vi "AB_Engine_RESTful_Verify_Configuration.vi"(6 "destinations":refnum<class "AB_Destination.lvclass">[](array[class]), 7 "path":path, 8 "error in (no error)":errorcluster, 10 "flat file layout":bool, 11 "sourceItems":refnum<class "AB_Source.lvclass">[](array[class])) -> (0 "error out":errorcluster, 1 "viConfigs":T1[](array[typedef]), 4 "relative VI paths":path[](array[path]))   [LabVIEW 2020]
uses:
  <vilib>/AppBuilder/AB_Classes/Source/AB_Source.lvclass
  <vilib>/AppBuilder/AB_Classes/Source/RESTfulVI/Configure_RESTfulVI/AB_RESTful_Configuration.ctl
  <vilib>/AppBuilder/AB_Classes/Source/RESTfulVI/Configure_RESTfulVI/AB_RESTful_VIType.ctl
  <vilib>/AppBuilder/AB_Classes/Source/RESTfulVI/Configure_RESTfulVI/AB_RESTful_OutputType.ctl
  <vilib>/AppBuilder/AB_Classes/Source/RESTfulVI/Configure_RESTfulVI/AB_RESTful_OutputFormat.ctl
  <vilib>/AppBuilder/AB_Classes/Destination/AB_Destination.lvclass
  <vilib>/AppBuilder/AB_Classes/Source/RESTfulVI/AB_Source_RESTfulVI.lvclass
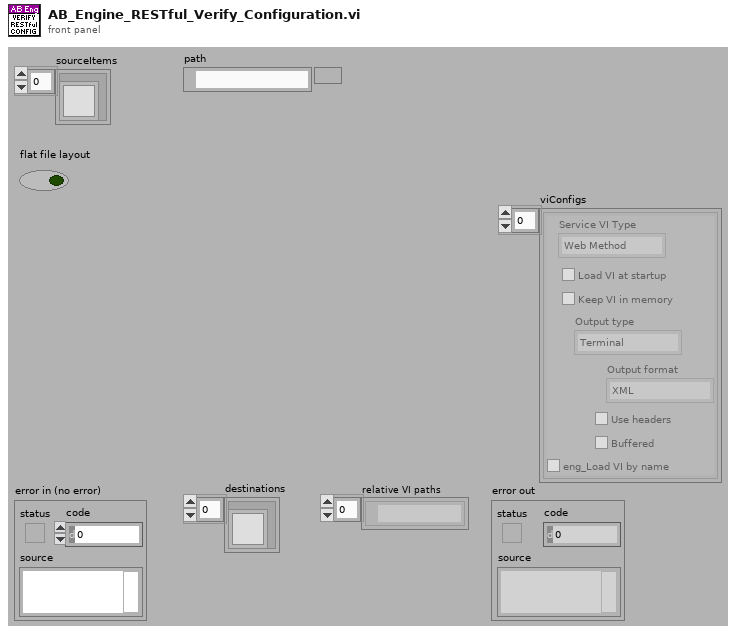
[diagram p1: front panel]
types:
  T1 = typedef "AB_RESTful_Configuration.ctl" = cluster{"Service VI Type":T2, "Load VI at statup":bool, "Keep VI in memory":bool, "Output type":T3, "Output format":T4, "Use headers":bool, "Buffered":bool, "eng_Load VI by name":bool}
  T2 = typedef "AB_RESTful_VIType.ctl" = enum32{"Web Method", "Auxiliary", "eng_Internal", "eng_Content"}
  T3 = typedef "AB_RESTful_OutputType.ctl" = enum32{"Terminal", "Stream"}
  T4 = typedef "AB_RESTful_OutputFormat.ctl" = enum32{"XML", "Text", "HTML", "JSON"}
  T5 = typedef "AB_Source.ctl" = cluster{"path":path, "itemID":string, "parentIndex":i32, "sourceInclusion":T6, "destinationIndex":i32, "properties":T7[], "newName":string, "lvfile":bool, "valid":bool, "eng_inBuild":bool, "eng_isNonVILink":bool, "Amalgamation":bool, "Amalgamation Piece":bool, "eng_delimitedName":string, "preventRename":bool}
  T6 = typedef "AB_Source_Inclusion.ctl" = enum16{"IncludeIfReferenced", "Include", "Exclude", "TopLevel"}
  T7 = typedef "AB_Source_Properties.ctl" = cluster{"sourcePropertyType":T8, "value":variant}
  T8 = typedef "AB_Source_Property_Type.ctl" = enum16{"Remove block diagram", "Remove front panel", "Password", "Window has title bar", "Show menu bar", "Show vertical scroll bar", "Show horizontal scroll bar", "Show toolbar", "Show Abort button", "Show fp when called", "Window behavior", "Allow user to close window", "Window run-time position", "Run when opened", "Allow debugging", "Auto error handling", "Generate guard code", "Use stack variables", "Expression folding", "Integer only", "Inline subVI"}
  T9 = typedef "AB_Destination.ctl" = cluster{"destName":string, "path":path, "libraryName":string, "preserveHierarchy":bool, "eng_inBuild":bool, "eng_libraryReference":refnum<vi>, "eng_restictAddToNewLibrary":bool}
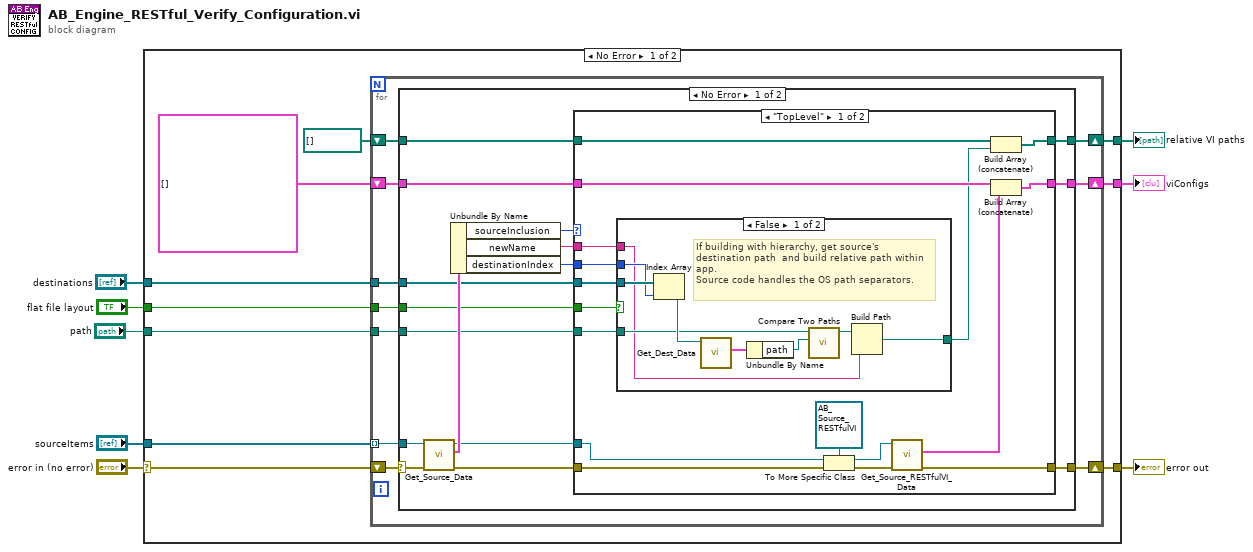
[diagram p0: block diagram]
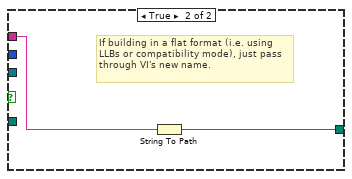
[diagram p2: hidden frame]
diagram:
  n1 = case shown="No Error" "error in (no error)" {
    selector: "error in (no error)" -> [w17 w79]
    tunnel: [w16 w79] -> w7
    tunnel: "sourceItems" -> [w18 _]
    tunnel: [w14 _] -> w5
    tunnel: "flat file layout" -> [w13 _]
    tunnel: "destinations" -> [w12 _]
    tunnel: "path" -> [w11 _]
    tunnel: [w9 _] -> w1
    frame No Error {
      n2 = for {
        tunnel: w18 -> [w28] mode=indexing
        shift-right: [w27] -> w16
        shift-left: w17 -> [w26]
        shift-right: [w25] -> w14
        shift-left: T1[] [] -> [w24]
        tunnel: w13 -> [w23]
        tunnel: w12 -> [w22]
        tunnel: w11 -> [w21]
        shift-right: [w20] -> w9
        shift-left: path[] [] -> [w19]
        n3 = case shown="No Error" w26 {
          selector: w26 -> [w37 w78]
          tunnel: w28 -> [w40 _]
          tunnel: [w38 w78] -> w27
          tunnel: [w36 w77] -> w25
          tunnel: w24 -> [w35 w77]
          tunnel: w23 -> [w34 _]
          tunnel: w22 -> [w32 _]
          tunnel: w21 -> [w31 _]
          tunnel: [w30 w76] -> w20
          tunnel: w19 -> [w29 w76]
          frame No Error {
            n4 = call <vilib>:"Get_Source_Data.vi"("error in (no error)"=w37, "Class in"=w40) -> ("error out"=w39:errorcluster, "data"=w44:T5, "Class out"=w41:refnum<class "AB_Source.lvclass">)  [unwired: 7 out]
            n5 = Unbundle By Name(w44) -> ("sourceInclusion"=w43:T6, "newName"=w42:string, "destinationIndex"=w33:i32)
            n6 = case shown="\"TopLevel\"" w43 {
              tunnel: w42 -> [w48 _]
              tunnel: w41 -> [w60 _]
              tunnel: w39 -> [w57 w75]
              tunnel: [w56 w75] -> w38
              tunnel: [w59 w74] -> w36
              tunnel: w35 -> [w58 w74]
              tunnel: w34 -> [w53 _]
              tunnel: w33 -> [w54 _]
              tunnel: w32 -> [w52 _]
              tunnel: w31 -> [w51 _]
              tunnel: [w46 w73] -> w30
              tunnel: w29 -> [w45 w73]
              frame "TopLevel" {
                n7 = case shown="False" w53 {
                  tunnel: w48 -> [w63 w72]
                  tunnel: [w62 w71] -> w47
                  tunnel: w52 -> [w70 _]
                  tunnel: w51 -> [w66 _]
                  tunnel: w54 -> [w69 _]
                  frame False {
                    # "If building with hierarchy, get source's destination path  and build relative path within app. \nSource code handles the OS path separators."
                    n8 = Index Array(array=w70, index=w69) -> (element=w68:refnum<class "AB_Destination.lvclass">)
                    n9 = call <vilib>:"Get_Dest_Data.vi"("Class in"=w68) -> ("destName"=w67:T9)  [unwired: 1 in, 9 out]
                    n10 = Unbundle By Name(w67) -> ("path"=w65:path)
                    n11 = call <vilib>:"Compare Two Paths.vi"("Path 2"=w65, "Path 1"=w66) -> ("Relative Path from 1 to 2"=w64:path)  [unwired: 1 in, 8 out]
                    n12 = Build Path(base path=w64, name or relative path=w63) -> (appended path=w62:path)
                  }
                  frame True {
                    # "If building in a flat format (i.e. using LLBs or compatibility mode), just pass through VI's new name."
                    n13 = String To Path(string=w72) -> (path=w71:path)
                  }
                }
                n14 = To More Specific Class(target class=refnum<class "AB_Source_RESTfulVI.lvclass"> refnum ("Class in"), reference=w60, error in=w57) -> (specific class reference=w50:refnum<class "AB_Source_RESTfulVI.lvclass">, error out=w49:errorcluster)
                n15 = call <vilib>:"Get_Source_RESTfulVI_Data.vi"("error in (no error)"=w49, "Class in"=w50) -> ("error out"=w56:errorcluster, "RESTful VI configuration"=w55:T1)  [unwired: 8 out]
                n16 = Build Array (concatenate)(w45, w47) -> (w46:path[])
                n17 = Build Array (concatenate)(w58, w55) -> (w59:T1[])
              }
              frame Default {
              }
            }
          }
          frame Error {
          }
        }
      }
    }
    frame Error {
    }
  }
  "error out" <- w7
  "viConfigs" <- w5
  "relative VI paths" <- w1
